vi "Run Integrator.vi"(8 "error in (no error)":errorcluster, 9 "Reset/Stop Integrator (False)":bool=TRUE, 10 "Enable Integrator (False)":bool=TRUE, 11 "VISA resource name":refnum<visa-resource-name>) -> (0 "error out":errorcluster, 3 "VISA resource name out":refnum<visa-resource-name>)   [LabVIEW 2015, in "Voltech PM1000+.lvlib"]
doc: "Start, stop or reset the PM1000+ integrator in order to measure Hrs, Whr, VAhr measurement items and so on. This vi is used when PM1000+ is set to Integrator mode by using \"Configure Mode\" vi.\n\n<b>Note:</b> Use of the \"Reset\" key to reset the PM1000+ integrator requires the integrator to be stopped first."
uses:
  <instrlib>/Voltech PM1000+/Voltech PM1000+.lvlib
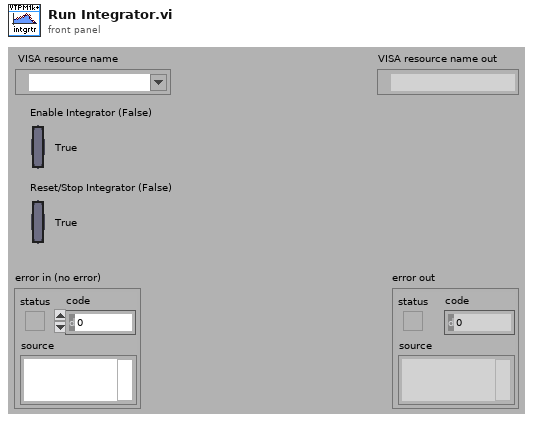
[diagram p1: front panel]
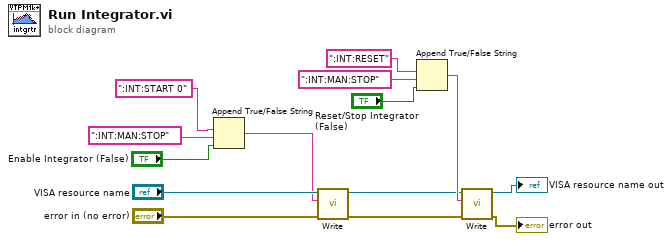
[diagram p0: block diagram]
diagram:
  n1 = Append True/False String(1:"Enable Integrator (False)", 2:":INT:MAN:STOP", 3:":INT:START 0") -> (0:w7:string)  [unwired: 1 in]
  n2 = call <instrlib>:"Write.vi"("error in (no error)"="error in (no error)", "Write Buffer"=w7, "VISA resource name"="VISA resource name") -> ("error out"=w3:errorcluster, "VISA resource name out"=w4:refnum<visa-resource-name>)  [unwired: 7 in]
  n3 = Append True/False String(1:"Reset/Stop Integrator (False)", 2:":INT:MAN:STOP", 3:":INT:RESET" ("multi-line string")) -> (0:w6:string)  [unwired: 1 in]
  n4 = call <instrlib>:"Write.vi"("error in (no error)"=w3, "Write Buffer"=w6, "VISA resource name"=w4) -> ("error out"=→"error out":errorcluster, "VISA resource name out"=→"VISA resource name out":refnum<visa-resource-name>)  [unwired: 7 in]
